vi "Template_Engine.vi"() -> ()   [LabVIEW 2013]
uses:
  Engine_VIs/enum_states.ctl
  <vilib>/httpClient/PUTBuffer.vi
  <vilib>/httpClient/LabVIEWHTTPClient.lvlib
panel:
  in  "JSON - PUT experiment":T1
  out "expResult":string
  out "Datavector Array":string[](array[string])
  out "Output Array":variant[](array[variant])
  out "Input Array":variant[](array[variant])
  out "expSpecification":string
  in  "JSON - GET experiment":T2
  out "Current State":T3
  out "request headers 2":string
  out "request body 2":string
  in  "error":errorcluster
  in  "config data":T4
  in  "stop":bool
  in  "JSON - GET status":T5
  out "request body":string
  out "request headers":string
  out "error out":errorcluster
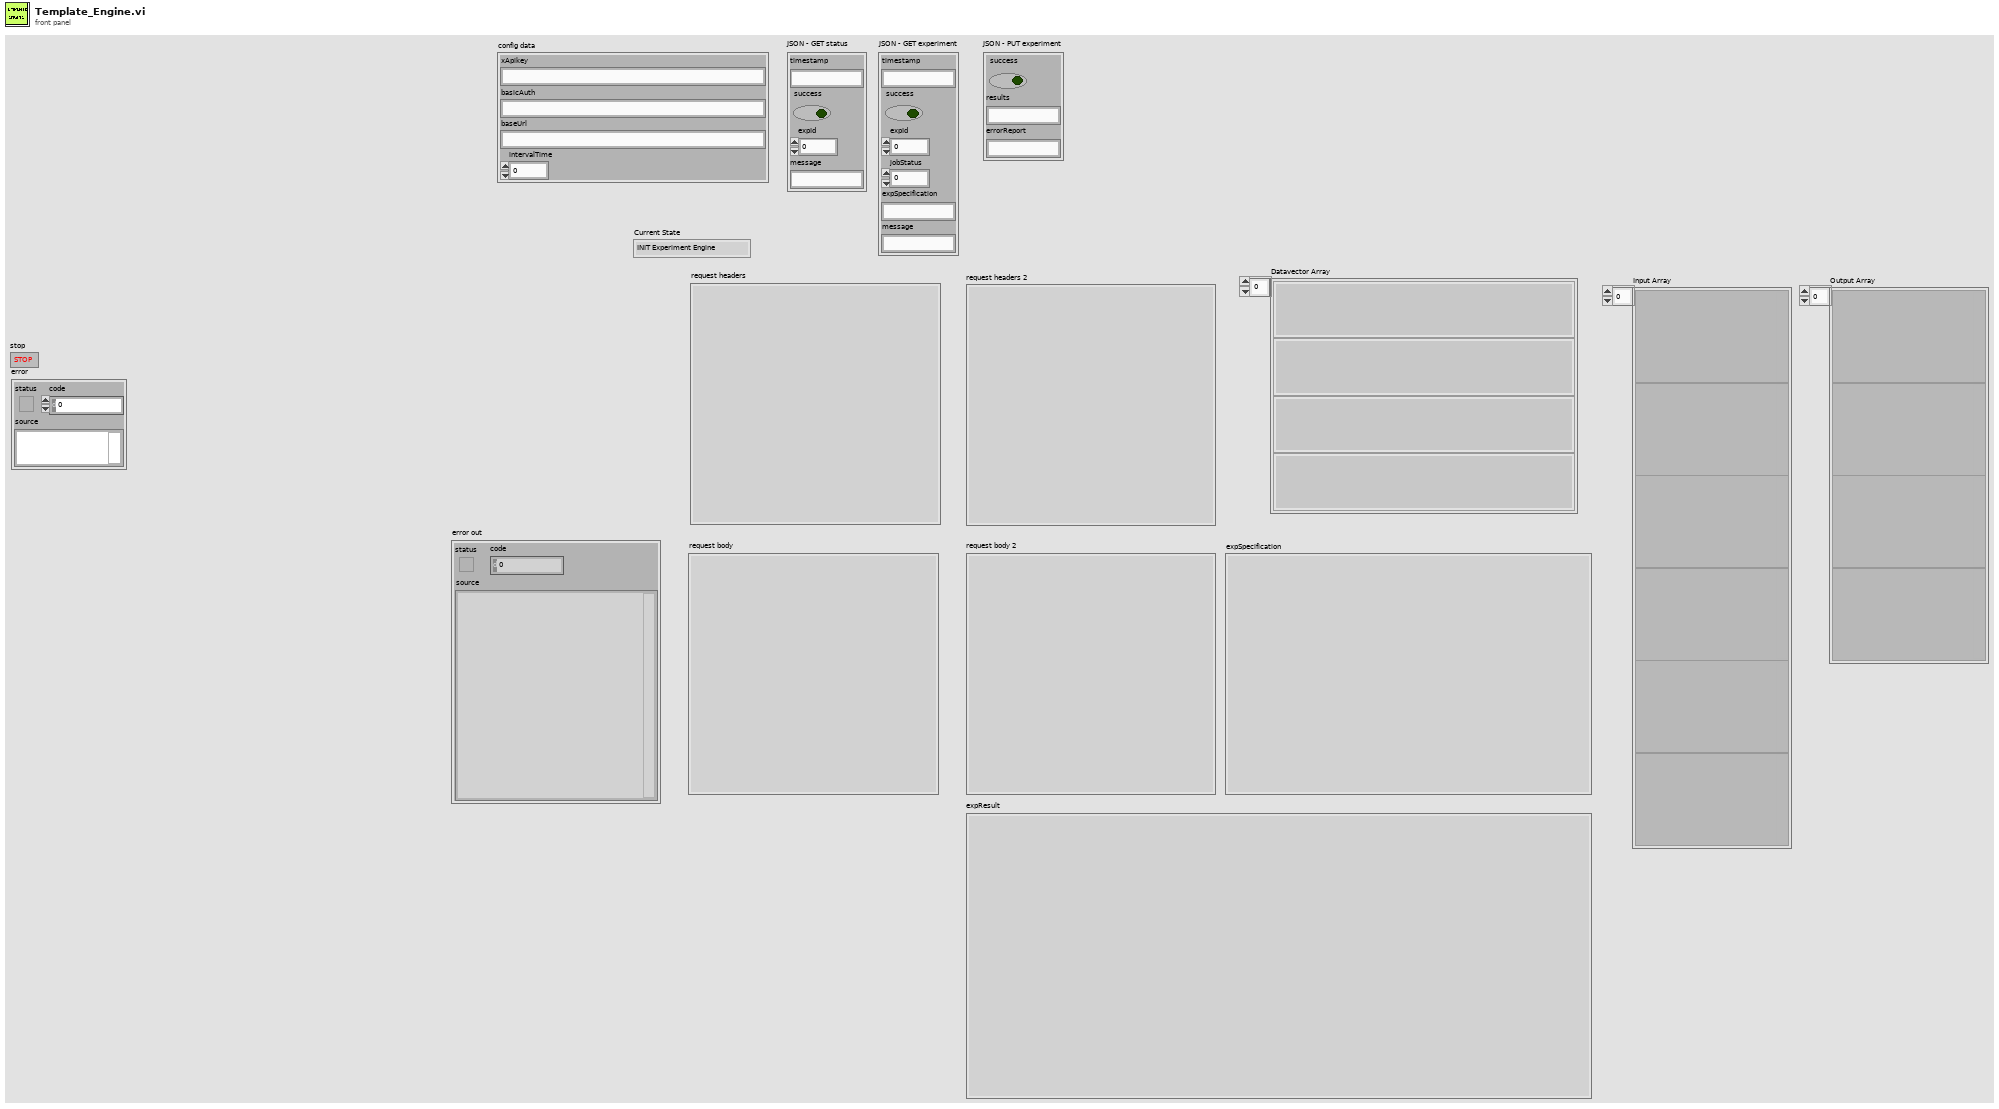
[diagram p1: front panel]
types:
  T1 = cluster{"success":bool, "results":string, "errorReport":string}
  T2 = cluster{"timestamp":string, "success":bool, "expId":i32, "jobStatus":i32, "expSpecification":string, "message":string}
  T3 = typedef "enum_states.ctl" = enum16{"INIT Experiment Engine", "REST - GET status", "REST - GET experiment", "PARSE ExpSpec", "RUN Experiment", "ASSEMBLE ExpResult", "REST - PUT experiment", "STOP"}
  T4 = cluster{"xApikey":string, "basicAuth":string, "baseUrl":string, "intervalTime":u32}
  T5 = cluster{"timestamp":string, "success":bool, "expId":i32, "message":string}
  T6 = cluster{"xApikey":string, "basicAuth":string, "baseUrl":string, "intervalTime":i32}
  T7 = typedef "LabVIEWHTTPClient.lvlib/ClientHandle.ctl" = refnum<k1>
  T8 = cluster{"parameter":string, "type info":string}[]
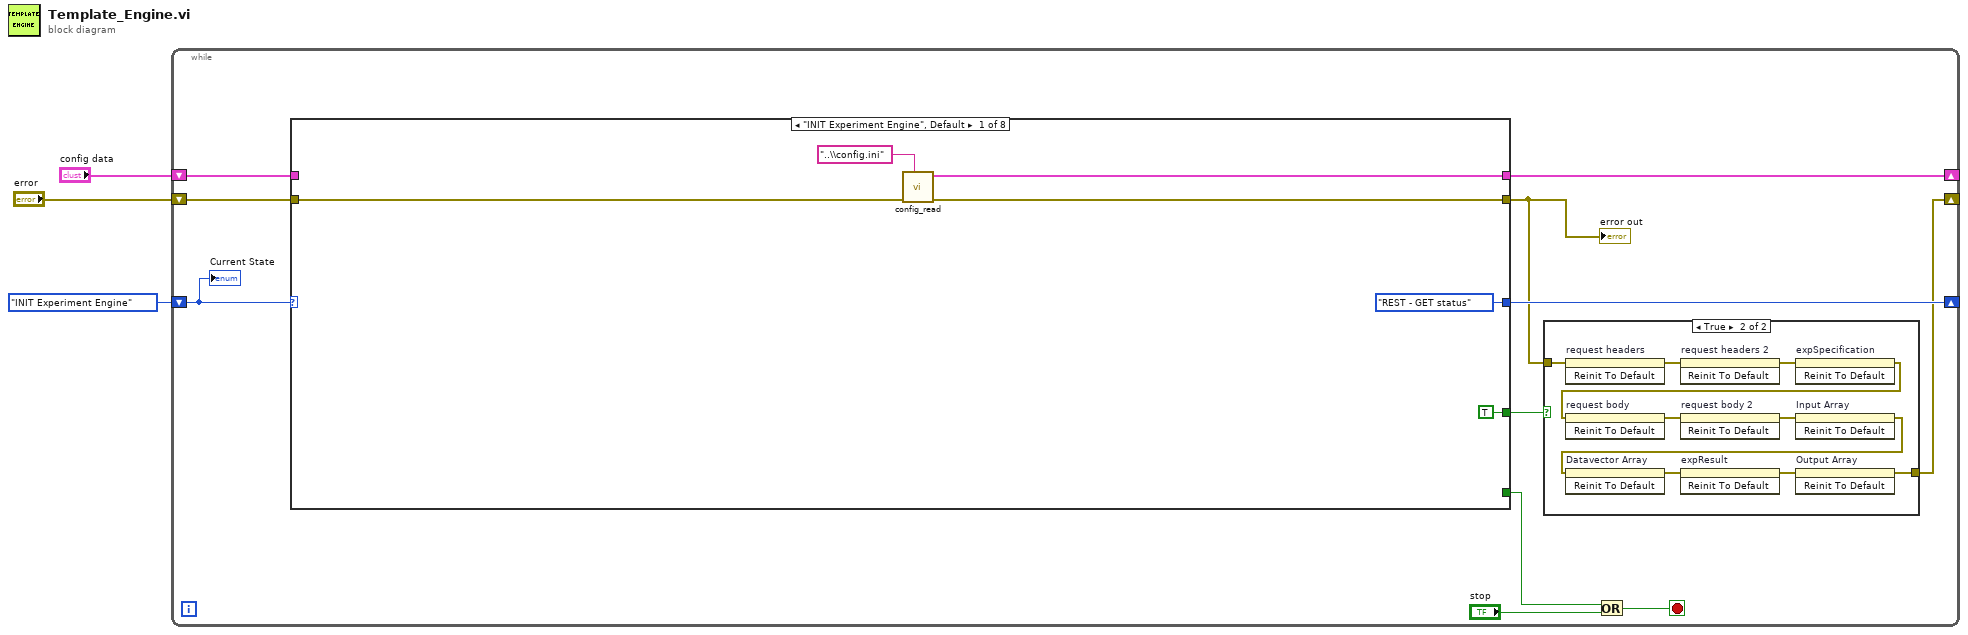
[diagram p0: block diagram]
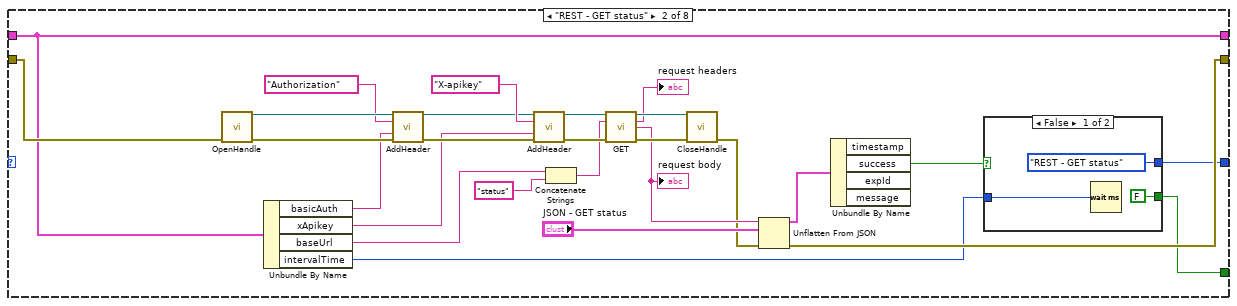
[diagram p3: hidden frame]
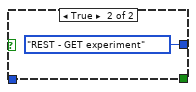
[diagram p4: hidden frame]
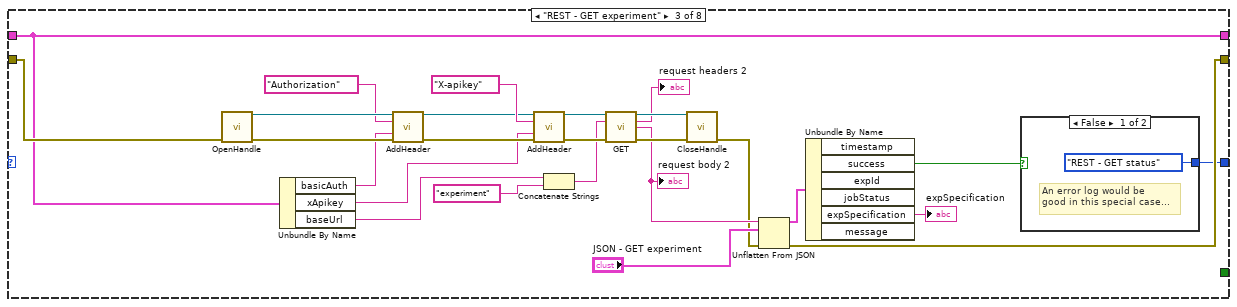
[diagram p5: hidden frame]
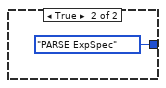
[diagram p6: hidden frame]
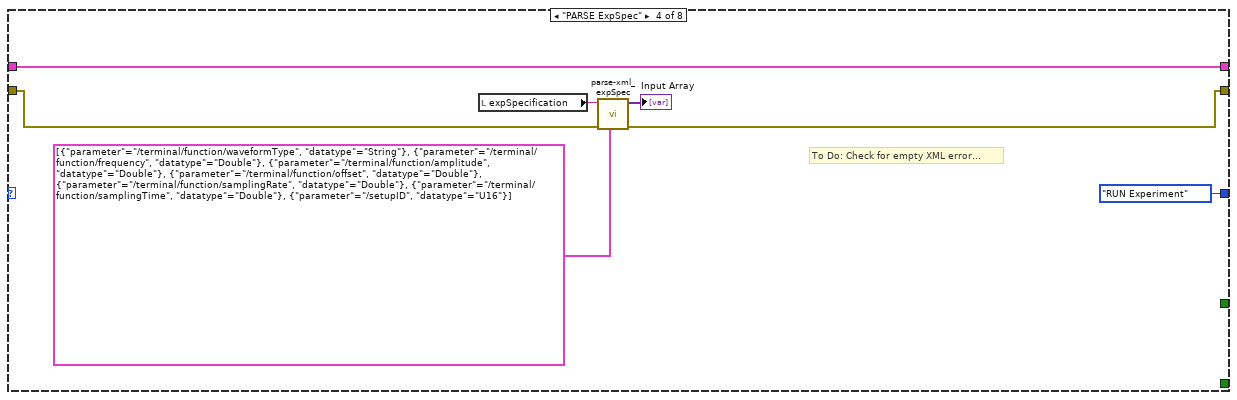
[diagram p7: hidden frame]
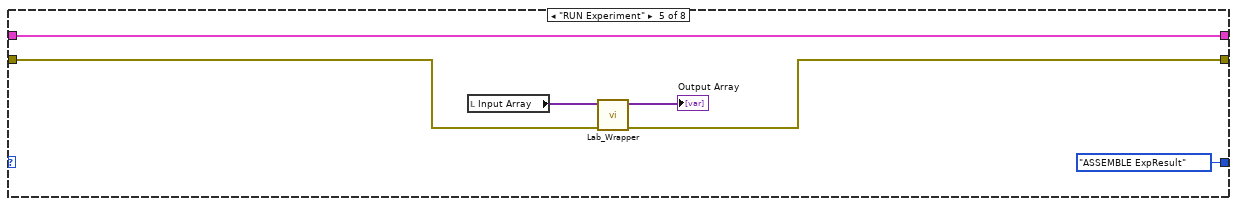
[diagram p8: hidden frame]
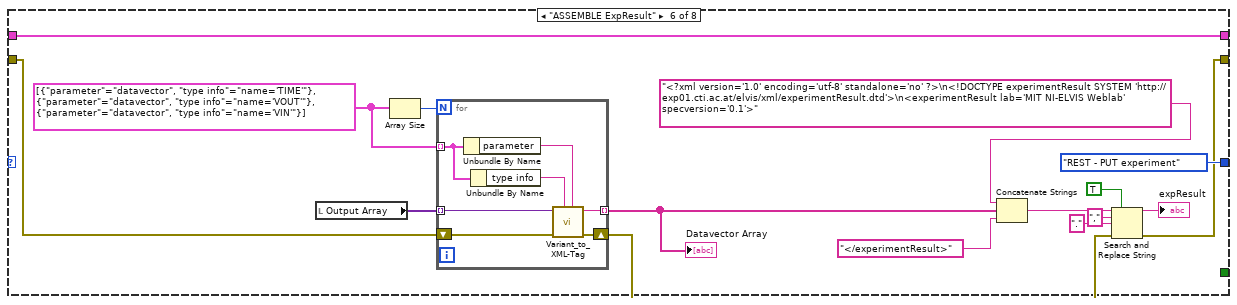
[diagram p9: hidden frame]
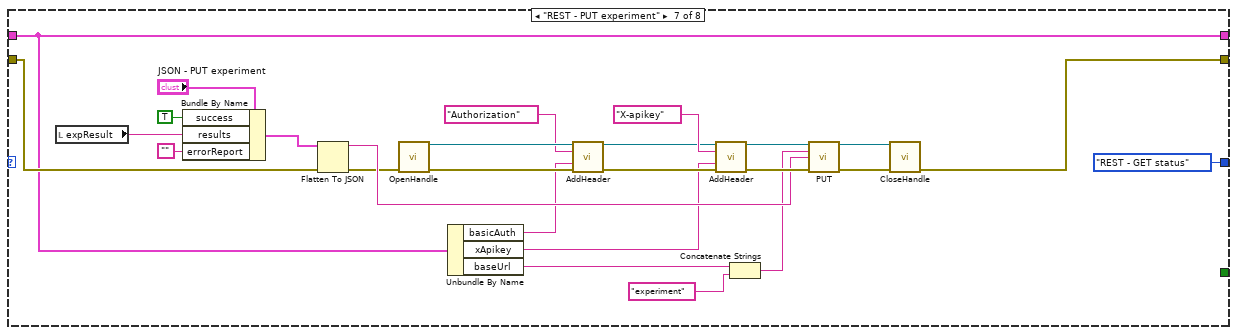
[diagram p10: hidden frame]
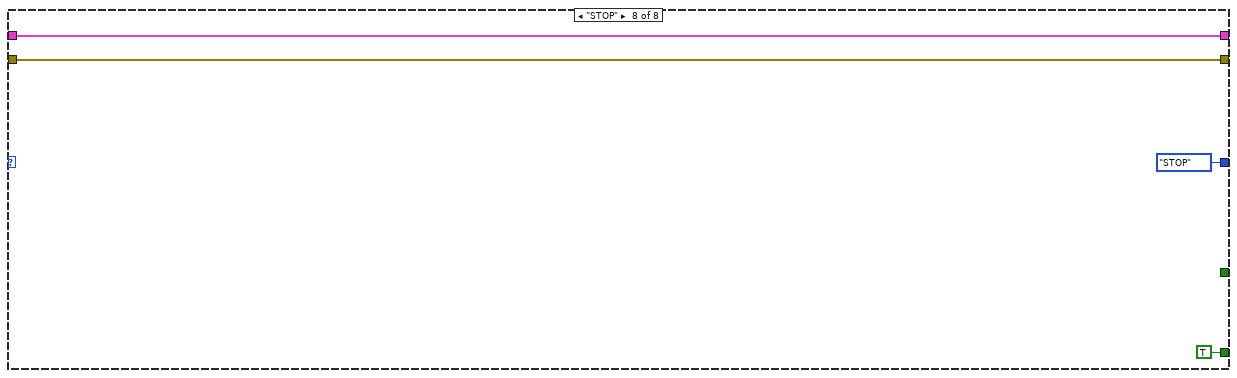
[diagram p11: hidden frame]
diagram:
  n1 = while {
    shift-right: [w13] -> _
    shift-left: enum_states."INIT Experiment Engine" ("states") -> [w14]
    shift-right: [w10] -> _
    shift-left: "config data" -> [w8]
    shift-right: [w4] -> _
    shift-left: "error" -> [w9]
    stop <- w12 stop-if-true
    n2 = case shown="\"INIT Experiment Engine\", Default" w14 {
      tunnel: [enum_states."REST - GET status" ("states") w41 w71 enum_states."RUN Experiment" ("states") enum_states."ASSEMBLE ExpResult" ("states") enum_states."REST - PUT experiment" ("states") enum_states."REST - GET status" ("states") enum_states."STOP" ("states")] -> w13
      tunnel: [w30 w38 w68 w97 w103 w118 w132 w155] -> w10
      tunnel: w9 -> [w29 w40 w69 w94 w99 w111 w134 w153]
      tunnel: w8 -> [_ w38 w68 w97 w103 w118 w132 w155]
      tunnel: [w28 w43 w75 w93 w98 w108 w133 w153] -> w5
      tunnel: [_ _ _ _ _ _ _ TRUE ("x")] -> w7
      tunnel: [TRUE w39 _ _ _ _ _ _] -> w6
      frame "INIT Experiment Engine", Default {
        n3 = call "config_read.vi"("name or relative path"="..\\config.ini", "error in (no error)"=w29) -> ("error out"=w28:errorcluster, "config data"=w30:T6)  [unwired: 8 in]
      }
      frame "REST - GET status" {
        n4 = call <vilib>:"OpenHandle.vi"("error in (no error)"=w40) -> ("client handle out"=w58:T7, "error out"=w57:errorcluster)  [unwired: 13 in]
        n5 = Unbundle By Name(w38) -> ("basicAuth"=w34:string, "xApikey"=w33:string, "baseUrl"=w35:string, "intervalTime"=w32:u32)
        n6 = call <vilib>:"AddHeader.vi"("client handle"=w58, "header"="Authorization", "value"=w34, "error in (no error)"=w57) -> ("client handle out"=w54:T7, "error out"=w53:errorcluster)  [unwired: 10 in]
        n7 = call <vilib>:"AddHeader.vi"("client handle"=w54, "header"="X-apikey", "value"=w33, "error in (no error)"=w53) -> ("client handle out"=w52:T7, "error out"=w51:errorcluster)  [unwired: 10 in]
        n8 = Concatenate Strings(w35, "status" ("url")) -> (w37:string)
        n9 = call <vilib>:"GET.vi"("client handle"=w52, "url"=w37, "error in (no error)"=w51) -> ("client handle out"=w50:T7, "headers"=→"request headers":string, "body"=w47:string, "error out"=w49:errorcluster)  [unwired: 9 in]
        "request body" <- w47
        n10 = call <vilib>:"CloseHandle.vi"("client handle"=w50, "error in (no error)"=w49) -> ("error out"=w45:errorcluster)  [unwired: 13 in]
        n11 = Unflatten From JSON(JSON string=w47, type and defaults="JSON - GET status", error in (no error)=w45) -> (value=w44:T5, error out=w43:errorcluster)  [unwired: 4 in]
        n12 = Unbundle By Name(w44) -> ("success"=w42:bool)  [unwired: 3 out]
        n13 = case shown="False" w42 {
          tunnel: [enum_states."REST - GET status" ("states") enum_states."REST - GET experiment" ("states")] -> w41
          tunnel: [FALSE _] -> w39
          tunnel: w32 -> [w59 _]
          frame False {
            n14 = Wait (ms)(milliseconds to wait=w59) -> ()  [unwired: 1 out]
          }
          frame True {
          }
        }
      }
      frame "REST - GET experiment" {
        n15 = call <vilib>:"OpenHandle.vi"("error in (no error)"=w69) -> ("client handle out"=w88:T7, "error out"=w87:errorcluster)  [unwired: 13 in]
        n16 = Unbundle By Name(w68) -> ("basicAuth"=w63:string, "xApikey"=w64:string, "baseUrl"=w65:string)
        n17 = call <vilib>:"AddHeader.vi"("client handle"=w88, "header"="Authorization", "value"=w63, "error in (no error)"=w87) -> ("client handle out"=w84:T7, "error out"=w83:errorcluster)  [unwired: 10 in]
        n18 = call <vilib>:"AddHeader.vi"("client handle"=w84, "header"="X-apikey", "value"=w64, "error in (no error)"=w83) -> ("client handle out"=w82:T7, "error out"=w81:errorcluster)  [unwired: 10 in]
        n19 = Concatenate Strings(w65, "experiment" ("url")) -> (w67:string)
        n20 = call <vilib>:"GET.vi"("client handle"=w82, "url"=w67, "error in (no error)"=w81) -> ("client handle out"=w80:T7, "headers"=→"request headers 2":string, "body"=w76:string, "error out"=w79:errorcluster)  [unwired: 9 in]
        "request body 2" <- w76
        n21 = call <vilib>:"CloseHandle.vi"("client handle"=w80, "error in (no error)"=w79) -> ("error out"=w74:errorcluster)  [unwired: 13 in]
        n22 = Unflatten From JSON(JSON string=w76, type and defaults="JSON - GET experiment", error in (no error)=w74) -> (value=w73:T2, error out=w75:errorcluster)  [unwired: 4 in]
        n23 = Unbundle By Name(w73) -> ("success"=w70:bool, "expSpecification"=→"expSpecification":string)  [unwired: 4 out]
        n24 = case shown="False" w70 {
          tunnel: [enum_states."REST - GET status" ("states") enum_states."PARSE ExpSpec" ("states")] -> w71
          frame False {
            # "An error log would be\ngood in this special case..."
          }
          frame True {
          }
        }
      }
      frame "PARSE ExpSpec" {
        # "To Do: Check for empty XML error..."
        n25 = local read "expSpecification"() -> (w95:string)
        n26 = call "parse-xml_expSpec.vi"("expSpecification XPath"=cluster{"parameter":string, "datatype":string}[] [{"parameter"="/terminal/function/waveformType", "datatype"="String"}, {"parameter"="/terminal/function/frequency", "datatype"="Double"}, {"parameter"="/terminal/function/amplitude", "datatype"="Double"}, {"parameter"="/terminal/function/offset", "datatype"="Double"}, {"parameter"="/terminal/function/samplingRate", "datatype"="Double"}, {"parameter"="/terminal/function/samplingTime", "datatype"="Double"}, {"parameter"="/setupID", "datatype"="U16"}], "error in (no error)"=w94, "expSpecification XML-String"=w95) -> ("error out"=w93:errorcluster, "Input Array"=→"Input Array":variant[])  [unwired: 7 in]
      }
      frame "RUN Experiment" {
        n27 = local read "Input Array"() -> (w100:variant[])
        n28 = call "Lab_Wrapper.vi"("error in (no error)"=w99, "Input Array"=w100) -> ("error out"=w98:errorcluster, "Output Array"=→"Output Array":variant[])  [unwired: 8 in]
      }
      frame "ASSEMBLE ExpResult" {
        w116 = T8 [{"parameter"="datavector", "type info"="name='TIME'"}, {"parameter"="datavector", "type info"="name='VOUT'"}, {"parameter"="datavector", "type info"="name='VIN'"}] ("Parameter out 2")
        n29 = local read "Output Array"() -> (w115:variant[])
        n30 = Array Size(array=w116) -> (size(s)=w117:i32)
        n31 = for {
          N: w117 -> [_]
          tunnel: w116 -> [w126] mode=indexing
          tunnel: [w123] -> w114 mode=indexing
          tunnel: w115 -> [w122] mode=indexing
          shift-right: [w120] -> w107
          shift-left: w111 -> [w121]
          n32 = Unbundle By Name(w126) -> ("parameter"=w124:string)
          n33 = Unbundle By Name(w126) -> ("type info"=w125:string)
          n34 = call "Variant_to_XML-Tag.vi"("parameter"=w124, "type info"=w125, "error in (no error)"=w121, "variant"=w122) -> ("error out"=w120:errorcluster, "XML tag"=w123:string)  [unwired: 6 in]
        }
        "Datavector Array" <- w114
        n35 = Concatenate Strings("<?xml version='1.0' encoding='utf-8' standalone='no' ?>\n<!DOCTYPE experimentResult SYSTEM 'http://exp01.cti.ac.at/elvis/xml/experimentResult.dtd'>\n<experimentResult lab='MIT NI-ELVIS Weblab' specversion='0.1'>", w114, "</experimentResult>") -> (w110:string)
        n36 = Search and Replace String(replace all?=TRUE ("replace all? (F)"), input string=w110, search string=",", replace string="." ("replace string (\"\")"), error in=w107) -> (result string=→"expResult":string, error out=w108:errorcluster)  [unwired: 3 in, 2 out]
      }
      frame "REST - PUT experiment" {
        n37 = local read "expResult"() -> (w138:string)
        n38 = Bundle By Name(cluster="JSON - PUT experiment", "success"=TRUE, "results"=w138, "errorReport"="") -> (w140:T1)
        n39 = Flatten To JSON(anything=w140, error in (no error)=w134) -> (JSON string=w139:string, 11:w135:errorcluster)  [unwired: 1 in]
        n40 = call <vilib>:"OpenHandle.vi"("error in (no error)"=w135) -> ("client handle out"=w151:T7, "error out"=w150:errorcluster)  [unwired: 13 in]
        n41 = Unbundle By Name(w132) -> ("basicAuth"=w129:string, "xApikey"=w128:string, "baseUrl"=w127:string)
        n42 = call <vilib>:"AddHeader.vi"("client handle"=w151, "header"="Authorization", "value"=w129, "error in (no error)"=w150) -> ("client handle out"=w147:T7, "error out"=w146:errorcluster)  [unwired: 10 in]
        n43 = call <vilib>:"AddHeader.vi"("client handle"=w147, "header"="X-apikey", "value"=w128, "error in (no error)"=w146) -> ("client handle out"=w145:T7, "error out"=w144:errorcluster)  [unwired: 10 in]
        n44 = Concatenate Strings(w127, "experiment" ("url")) -> (w130:string)
        n45 = call-poly <vilib>:"PUT.vi"("client handle"=w145, "url"=w130, "buffer"=w139, "error in (no error)"=w144) -> ("client handle out"=w143:T7, "error out"=w142:errorcluster)  [unwired: 8 in, 2 out]
        n46 = call <vilib>:"CloseHandle.vi"("client handle"=w143, "error in (no error)"=w142) -> ("error out"=w133:errorcluster)  [unwired: 13 in]
      }
      frame "STOP" {
      }
    }
    "error out" <- w5
    n47 = case shown="True" w6 {
      tunnel: w5 -> [w15 w17]
      tunnel: [w15 w16] -> w4
      frame False {
      }
      frame True {
        n48 = invoke on="request headers" class="Str" method="Reinit To Default"(error in=w17) -> (error out=w25:errorcluster)  [unwired: 2 in, 2 out]
        n49 = invoke on="request headers 2" class="Str" method="Reinit To Default"(error in=w25) -> (error out=w24:errorcluster)  [unwired: 2 in, 2 out]
        n50 = invoke on="expSpecification" class="Str" method="Reinit To Default"(error in=w24) -> (error out=w23:errorcluster)  [unwired: 2 in, 2 out]
        n51 = invoke on="request body" class="Str" method="Reinit To Default"(error in=w23) -> (error out=w21:errorcluster)  [unwired: 2 in, 2 out]
        n52 = invoke on="request body 2" class="Str" method="Reinit To Default"(error in=w21) -> (error out=w20:errorcluster)  [unwired: 2 in, 2 out]
        n53 = invoke on="Input Array" class="Arr (strict)" method="Reinit To Default"(error in=w20) -> (error out=w22:errorcluster)  [unwired: 2 in, 2 out]
        n54 = invoke on="Datavector Array" class="Arr (strict)" method="Reinit To Default"(error in=w22) -> (error out=w19:errorcluster)  [unwired: 2 in, 2 out]
        n55 = invoke on="expResult" class="Str" method="Reinit To Default"(error in=w19) -> (error out=w18:errorcluster)  [unwired: 2 in, 2 out]
        n56 = invoke on="Output Array" class="Arr (strict)" method="Reinit To Default"(error in=w18) -> (error out=w16:errorcluster)  [unwired: 2 in, 2 out]
      }
    }
    n57 = Or(x=w7, y="stop") -> (x .or. y?=w12:bool)
    "Current State" <- w14
  }
